vi "SubVI_Modbus.vi"(8 "error in (no error)":errorcluster, 11 "TCP Network Connection in":refnum<k5>) -> (0 "error out":errorcluster, 1 "Time has Elapsed":bool, 2 "Coils":bool[](array[boolean]), 3 "TCP Network Connection out":refnum<k5>)   [LabVIEW 2017]
uses:
  <vilib>/NI Modbus.llb/MB Ethernet Master Query Read Coils (poly).vi
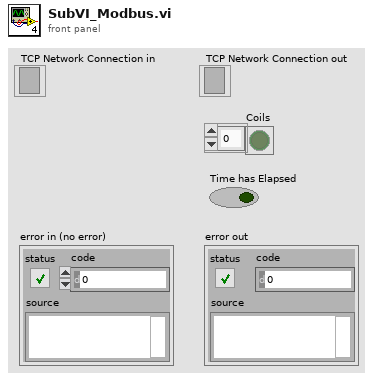
[diagram p1: front panel]
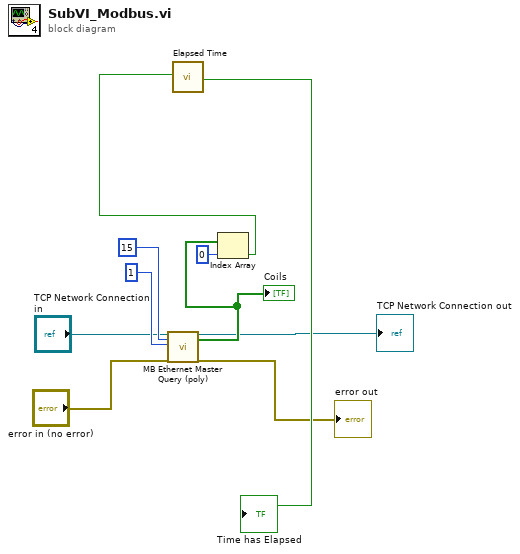
[diagram p0: block diagram]
diagram:
  n1 = call-poly <vilib>:"MB Ethernet Master Query (poly).vi"("TCP Connection Refnum in"="TCP Network Connection in", "Starting Address"=u16 15, "Quantity"=u16 1, "error in"="error in (no error)") -> ("TCP Connection Refnum (dup)"=→"TCP Network Connection out":refnum<k5>, "Coils"=w7:bool[], "error out"=→"error out":errorcluster)  [unwired: 12 in, 1 out]
  "Coils" <- w7
  n2 = Index Array(array=w7, index=0) -> (element=w9:bool)
  n3 = call "Elapsed Time"("Reset"=w9) -> ("Time has Elapsed"=→"Time has Elapsed":bool)  [unwired: 11 in, 7 out]
